vi "Wait Ready to Close.vi"(8 "error in (no error)":errorcluster, 9 "ignore previous (T)":bool, 10 "ms timeout (-1)":i32=-1, 11 "navX - Interface in":refnum<class "navX - Interface.lvclass">) -> (0 "error out":errorcluster, 1 "timed out":bool, 3 "navX - Interface out":refnum<class "navX - Interface.lvclass">)   [LabVIEW 2015, in "navX Library v3.lvlib" / "navX - Interface.lvclass"]
uses:
  navX - Interface.lvclass
  navX - Interface.lvclass/navX - Interface.ctl
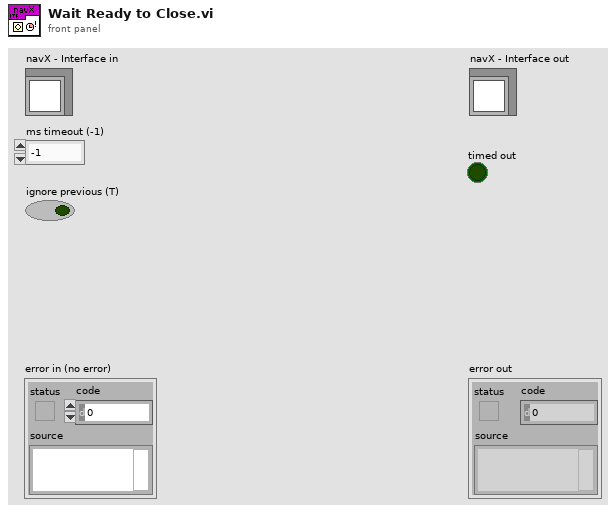
[diagram p1: front panel]
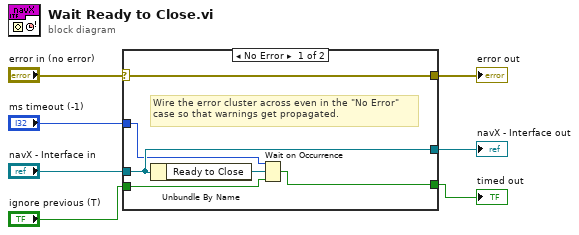
[diagram p0: block diagram]
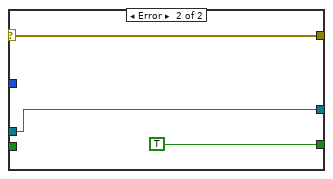
[diagram p2: hidden frame]
diagram:
  n1 = case shown="No Error" "error in (no error)" {
    selector: "error in (no error)" -> [w13 w16]
    tunnel: [w13 w16] -> w6
    tunnel: [w12 w15] -> w4
    tunnel: "navX - Interface in" -> [w12 w15]
    tunnel: "ignore previous (T)" -> [w10 _]
    tunnel: "ms timeout (-1)" -> [w9 _]
    tunnel: [w8 TRUE ("timed out")] -> w1
    frame No Error {
      # "Wire the error cluster across even in the \"No Error\"\ncase so that warnings get propagated."
      n2 = Unbundle By Name(w12) -> ("Ready to Close"=w11:refnum<k4>)
      n3 = Wait on Occurrence(1:w10, 2:w11, 3:w9) -> (0:w8:bool)
    }
    frame Error {
    }
  }
  "error out" <- w6
  "navX - Interface out" <- w4
  "timed out" <- w1
